vi "Check if VI Can Be Added.vi"(8 "error in":errorcluster, 9 "only accept open windows? (F)":bool, 10 "VIs to exclude":variant, 11 "VI refnum":refnum<vi>) -> (0 "error out":errorcluster, 3 "allowed?":bool)   [LabVIEW 2010, in "NI_SE_Config Front Panel Layout.lvlib"]
uses:
  NI_SE_Config Front Panel Layout.lvlib
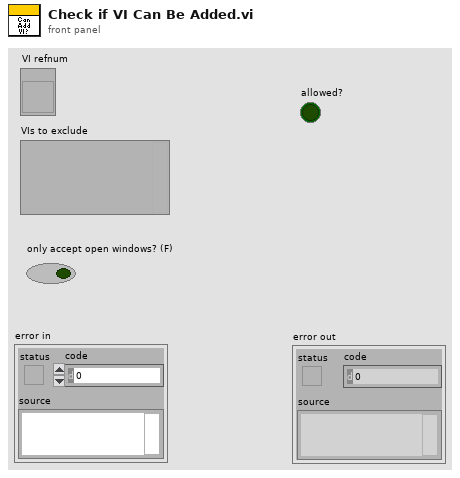
[diagram p1: front panel]
types:
  T1 = enum32{"Invalid", "Standard", "Closed", "Hidden", "Minimized", "Maximized"}
  T2 = enum32{"Bad", "Idle", "Run top level", "Running"}
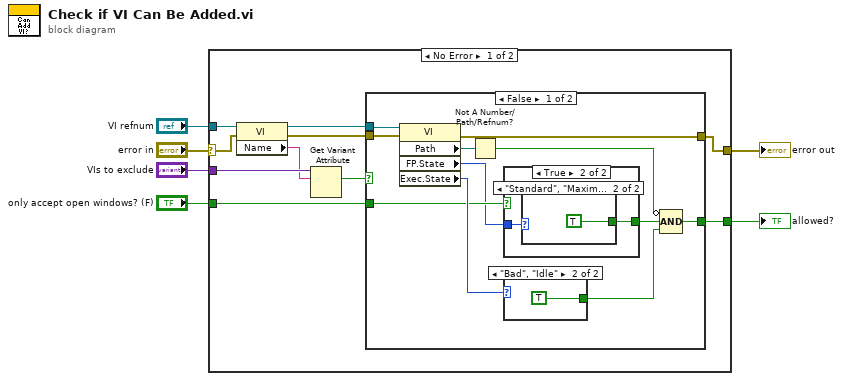
[diagram p0: block diagram]
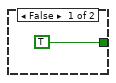
[diagram p2: hidden frame]
diagram:
  n1 = case shown="No Error" "error in" {
    selector: "error in" -> [w12 w34]
    tunnel: "VIs to exclude" -> [w16 _]
    tunnel: "VI refnum" -> [w15 _]
    tunnel: "only accept open windows? (F)" -> [w9 _]
    tunnel: [w8 w34] -> w2
    tunnel: [w7 _] -> w1
    frame No Error {
      n2 = property class="VI"(reference=w15, error in=w12) -> (reference out=w10:refnum<vi>, error out=w11:errorcluster, "Name"=w14:string)
      n3 = Get Variant Attribute(Variant=w16, name=w14) -> (found=w13:bool)  [unwired: 2 in, 3 out]
      n4 = case shown="False" w13 {
        tunnel: w11 -> [w26 w33]
        tunnel: w10 -> [w27 _]
        tunnel: w9 -> [w24 _]
        tunnel: [w21 w33] -> w8
        tunnel: [w20 _] -> w7
        frame False {
          n5 = property class="VI"(reference=w27, error in=w26) -> (error out=w21:errorcluster, "Path"=w18:path, "FP.State"=w19:T1, "Exec.State"=w25:T2)  [unwired: 1 out]
          n6 = Not A Number/Path/Refnum?(number/path/refnum=w18) -> (NaN/Path/Refnum?=w17:bool)
          n7 = case shown="True" w24 {
            tunnel: w19 -> [_ w30]
            tunnel: [TRUE w29] -> w23
            frame False {
            }
            frame True {
              n8 = case shown="\"Standard\", \"Maximized\"" w30 {
                tunnel: [_ TRUE] -> w29
                frame Default {
                }
                frame "Standard", "Maximized" {
                }
              }
            }
          }
          n9 = case shown="\"Bad\", \"Idle\"" w25 {
            tunnel: [_ TRUE] -> w22
            frame Default {
            }
            frame "Bad", "Idle" {
            }
          }
          n10 = Compound Arithmetic op=AND(invert w17, w23, w22) -> (w20:bool)
        }
        frame True {
        }
      }
    }
    frame Error {
    }
  }
  "error out" <- w2
  "allowed?" <- w1
